vi "_PC_SaveFile convMATFormat.vi"(7 "Matrix Name":string="dbl", 8 "error in (no error)":errorcluster, 10 "Data Array":dbl[](array[numeric]), 11 "path refnum in":refnum<file>) -> (0 "error out":errorcluster, 3 "path refnum out":refnum<file>)   [LabVIEW 2018]
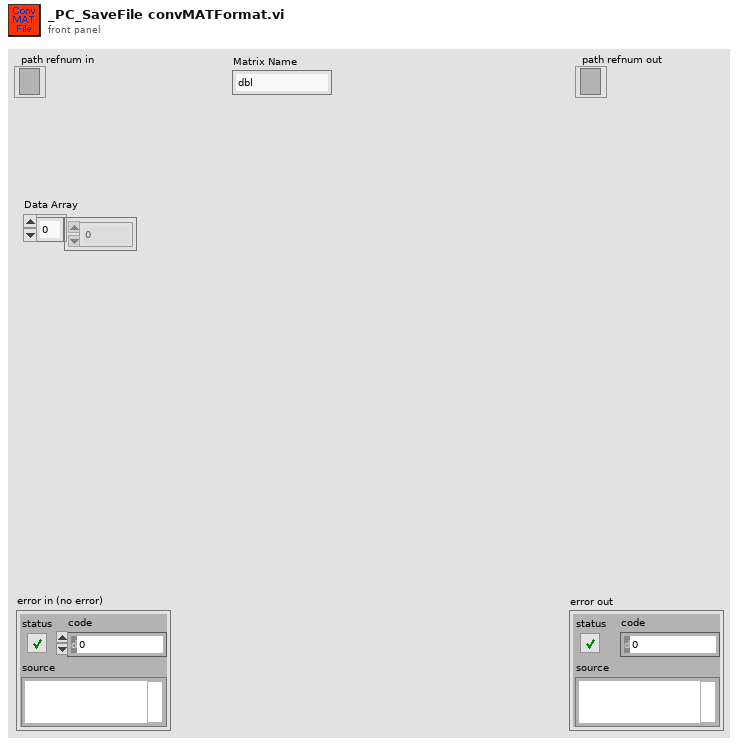
[diagram p1: front panel]
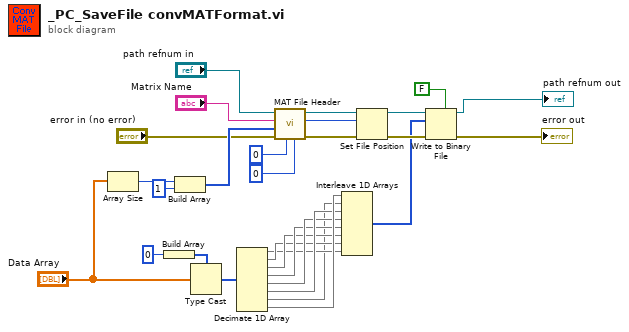
[diagram p0: block diagram]
diagram:
  n1 = Array Size(array="Data Array") -> (size(s)=w29:i32)
  n2 = Build Array(u8 0) -> (w18:u8[])
  n3 = Build Array(w29, 1 ("element")) -> (w13:i32[])
  n4 = Type Cast(type=w18, x="Data Array") -> (*(type *) &x=w17:u8[])
  n5 = Decimate 1D Array(w17) -> (w21:u8[], w22:u8[], w23:u8[], w24:u8[], w25:u8[], w26:u8[], w20:u8[], w27:u8[])
  n6 = call "MAT File Header"("Real/Complex (0-Real)"=u32 0, "Rep. Code"=u32 0, "error in (no error)"="error in (no error)", "Matrix Size"=w13, "Matrix Name"="Matrix Name", "Ref Num"="path refnum in") -> ("error out"=w9:errorcluster, "offset"=w8:i32, "Dup Ref Num"=w10:refnum<file>)  [unwired: 3 in]
  n7 = Interleave 1D Arrays(w27, w20, w26, w25, w24, w23, w22, w21) -> (w4:u8[])
  n8 = Set File Position(offset (in bytes) (0)=w8, refnum=w10, error in=w9) -> (refnum out=w6:refnum<file>, error out=w5:errorcluster)  [unwired: 1 in]
  n9 = Write to Binary File(file (use dialog)=w6, data=w4, error in=w5, 5:FALSE ("prepend array or string size? (T)")) -> (refnum out=→"path refnum out":refnum<file>, error out=→"error out":errorcluster)  [unwired: 2 in, 1 out]
